vi "Create Map of VI and Lib Ref.vi"(8 "error in":errorcluster caption="error out", 9 "Plugin OS":T1=enum."Env Server" caption="OS", 11 "VI and Library References":T2[](array[typedef])) -> (0 "error out":errorcluster, 2 "Map - LibRef":map{string, refnum<vi>}(c390), 3 "Map - VIRef":map{string, refnum<vi>}(c390))   [LabVIEW 2023, in "Plugin Generator.lvlib"]
uses:
  Plugin Generator.lvlib
  <vilib>/Utility/EditLVProj/Library And VI References.ctl
  Typedef/Plugin OS.ctl
  <vilib>/Utility/EditLVProj/Edit LVProj.lvlib
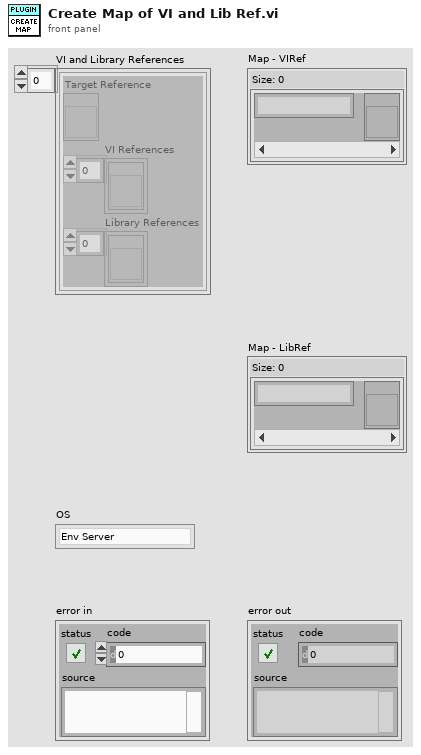
[diagram p1: front panel]
types:
  T1 = typedef "Plugin Generator.lvlib/Plugin OS.ctl" = enum16{"Linux RT", "Env Server"}
  T2 = typedef "Edit LVProj.lvlib/Library And VI References.ctl" = cluster{"Target Reference":refnum<vi>, "VI References":refnum<vi>[], "Library References":refnum<vi>[]}
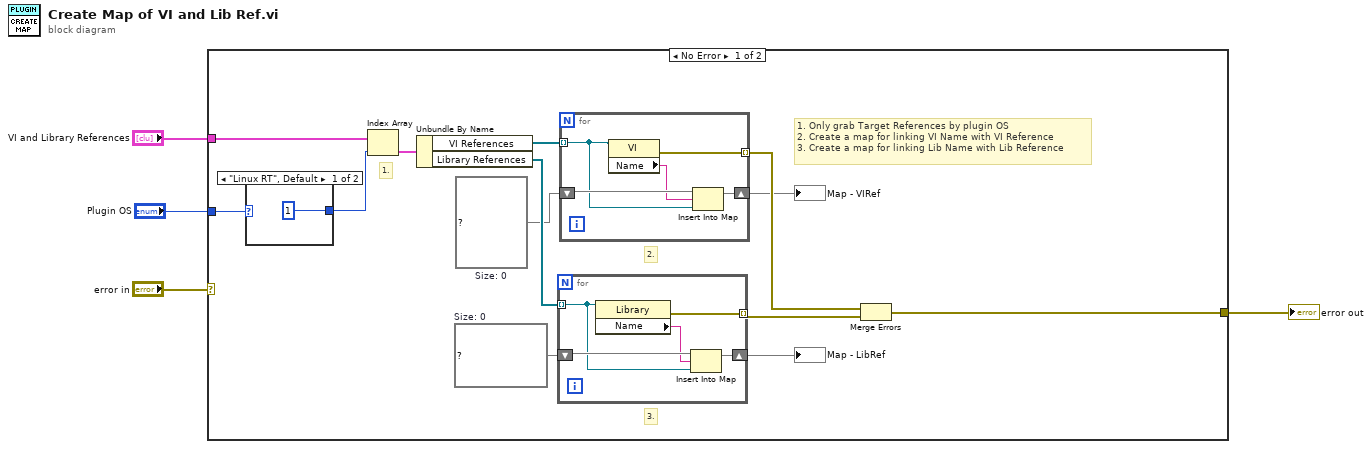
[diagram p0: block diagram]
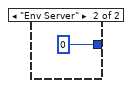
[diagram p2: hidden frame]
diagram:
  n1 = case shown="No Error" "error in" {
    selector: "error in" -> [_ w30]
    tunnel: "VI and Library References" -> [w15 _]
    tunnel: [w8 w30] -> w2
    tunnel: "Plugin OS" -> [w6 _]
    frame No Error {
      w11 = map{string, refnum<vi>} {}  # Size: 0
      w16 = map{string, refnum<vi>} {}  # Size: 0
      # "2."
      # "1."
      # "1. Only grab Target References by plugin OS\n2. Create a map for linking VI Name with VI Reference\n3. Create a map for linking Lib Name with Lib Reference"
      # "3."
      n2 = case shown="\"Linux RT\", Default" w6 {
        tunnel: [1 ("index") 0 ("index")] -> w5
        frame "Linux RT", Default {
        }
        frame "Env Server" {
        }
      }
      n3 = Index Array(array=w15, index=w5) -> (element=w14:T2)
      n4 = Unbundle By Name(w14) -> ("VI References"=w12:refnum<vi>[], "Library References"=w13:refnum<vi>[])
      n5 = for {
        shift-right: [w28] -> w17
        shift-left: w16 -> [w29]
        tunnel: w13 -> [w26] mode=indexing
        tunnel: [w25] -> w10 mode=indexing
        n6 = property class="Library"(reference=w26) -> (error out=w25:errorcluster, "Name"=w27:string)  [unwired: 1 in, 1 out]
        n7 = Insert Into Map(map in=w29, key=w27, value=w26) -> (map out=w28:map{string, refnum<vi>})  [unwired: 2 out]
      }
      "Map - LibRef" <- w17
      n8 = for {
        shift-right: [w23] -> w7
        shift-left: w11 -> [w24]
        tunnel: w12 -> [w22] mode=indexing
        tunnel: [w20] -> w9 mode=indexing
        n9 = property class="VI"(reference=w22) -> (error out=w20:errorcluster, "Name"=w21:string)  [unwired: 1 in, 1 out]
        n10 = Insert Into Map(map in=w24, key=w21, value=w22) -> (map out=w23:map{string, refnum<vi>})  [unwired: 2 out]
      }
      "Map - VIRef" <- w7
      n11 = Merge Errors(w9, w10) -> (w8:errorcluster)
    }
    frame Error {
    }
  }
  "error out" <- w2
